vi "SerialNo.vi"() -> (2 "Continue?":bool)   [LabVIEW 2019]
uses:
  globals/QC_RunInformation.vi
panel:
  in  "DB Serial No.:":string
  in  "Device Category:":string(combo)="ATLAS18SS"
  in  "Manufacturer:":string(combo)="Hamamatsu"
  in  "Sensor Serial No.:":string
  in  "Cancel":bool
  in  "OK":bool
  in  "Barcode reader":bool
  # "ATLAS Serial No."
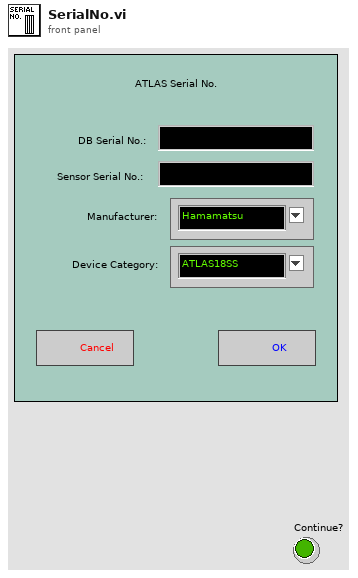
[diagram p1: front panel]
types:
  T1 = cluster{"Institute":string, "Manufacturers":string[], "Devices":string[], "Serialnumbers Lookup DB":string, "Data directory":string, "Backup & screenshot directory":string, "List of known users":string[], "Measurement switch not used":bool, "Measurement Switch":string, "DUT Switch":string}
  T2 = cluster{"Sensor Serial No.:":string, "Wafer Serial No.:":string, "Batch:":string, "Manufacturer:":string, "Device Category:":string, "Database Serial No.:":string, "Date Initiated:":string, "Time Initiated:":string, "Test":string, "Instruments used:":string, "Probeplan used:":string, "End of Run comment:":string, "User:":string}
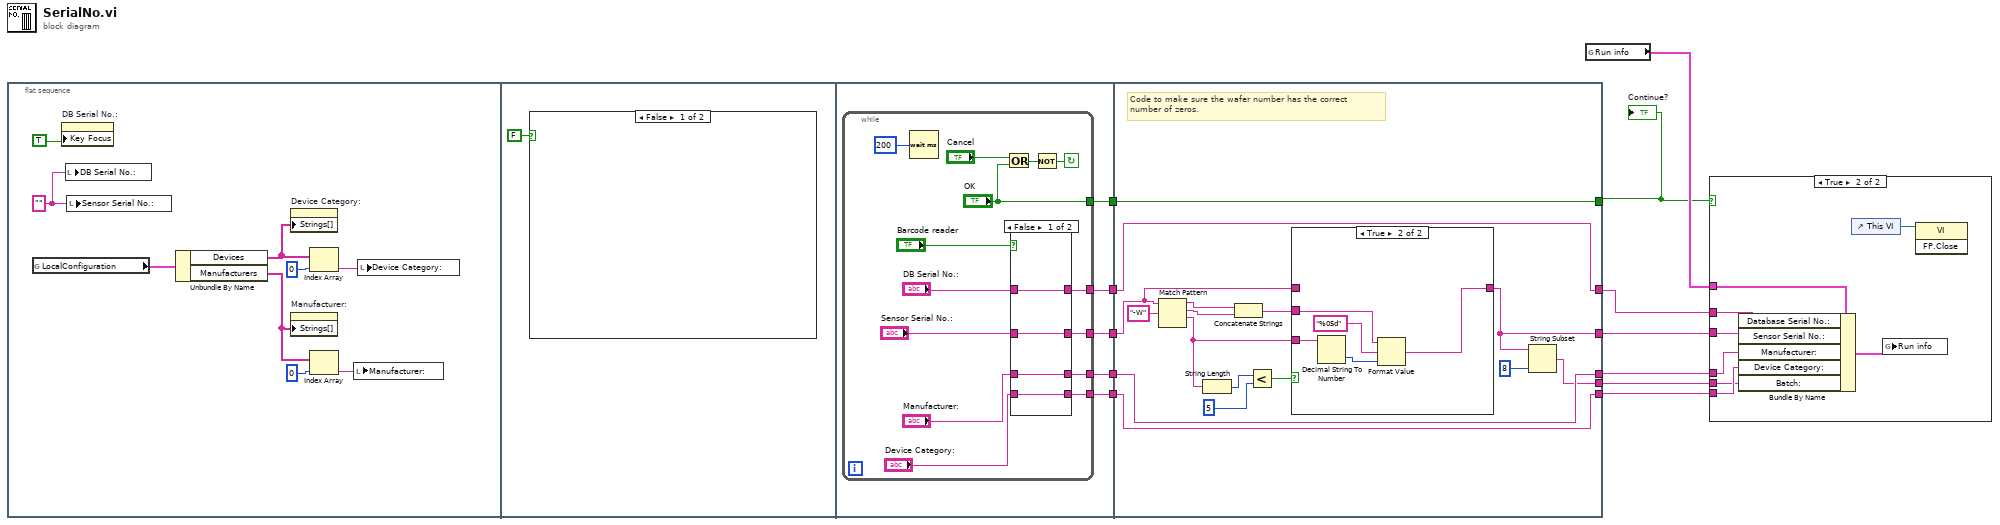
[diagram p0: block diagram]
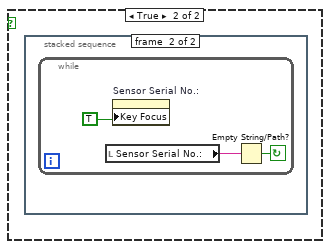
[diagram p3: hidden frame]
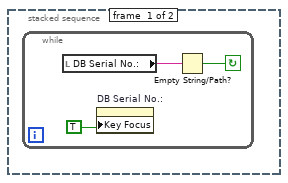
[diagram p4: hidden frame]
diagram:
  n1 = flat-sequence {
    tunnel: [w33] -> w7
    tunnel: [w32] -> w6
    tunnel: [w31] -> w5
    tunnel: [w30] -> w4
    tunnel: [w29] -> w3
    tunnel: [w68] -> w11
    tunnel: [w69] -> w10
    tunnel: [w70] -> w8
    tunnel: [w71] -> w12
    tunnel: w7 -> [w71]
    tunnel: w6 -> [w70]
    tunnel: w5 -> [w69]
    tunnel: w4 -> [w68]
    tunnel: w3 -> [w62]
    tunnel: [w58] -> w2
    tunnel: [w56] -> w1
    frame #0 {
      w21 = ""
      n2 = global read "QC_RunInformation.vi" "LocalConfiguration"() -> (w19:T1)
      n3 = property on="DB Serial No.:" class="Str"("Key Focus"=TRUE) -> ()  [unwired: 2 in, 2 out]
      n4 = local write "DB Serial No.:"(w21) -> ()
      n5 = local write "Sensor Serial No.:"(w21) -> ()
      n6 = Unbundle By Name(w19) -> ("Devices"=w14:string[], "Manufacturers"=w13:string[])
      n7 = property on="Device Category:" class="CmbBox"("Strings[]"=w14) -> ()  [unwired: 2 in, 2 out]
      n8 = property on="Manufacturer:" class="CmbBox"("Strings[]"=w13) -> ()  [unwired: 2 in, 2 out]
      n9 = Index Array(array=w14, index=0) -> (element=w15:string)
      n10 = Index Array(array=w13, index=0) -> (element=w16:string)
      n11 = local write "Manufacturer:"(w16) -> ()
      n12 = local write "Device Category:"(w15) -> ()
    }
    frame #1 {
      n13 = case shown="False" FALSE {
        frame False {
        }
        frame True {
          n14 = stacked-sequence {
            frame #0 {
              n15 = while {
                stop <- w23 continue-if-true
                n16 = local read "DB Serial No.:"() -> (w24:string)
                n17 = property on="DB Serial No.:" class="Str"("Key Focus"=TRUE) -> ()  [unwired: 2 in, 2 out]
                n18 = Empty String/Path?(string/path=w24) -> (empty?=w23:bool)
              }
            }
            frame #1 {
              n19 = while {
                stop <- w27 continue-if-true
                n20 = local read "Sensor Serial No.:"() -> (w26:string)
                n21 = property on="Sensor Serial No.:" class="Str"("Key Focus"=TRUE) -> ()  [unwired: 2 in, 2 out]
                n22 = Empty String/Path?(string/path=w26) -> (empty?=w27:bool)
              }
            }
          }
        }
      }
    }
    frame #2 {
      n23 = while {
        tunnel: ["OK"] -> w32
        tunnel: [w40] -> w29
        tunnel: [w41] -> w33
        tunnel: [w39] -> w31
        tunnel: [w38] -> w30
        stop <- w45 continue-if-true
        n24 = Wait (ms)(milliseconds to wait=200) -> ()  [unwired: 1 out]
        n25 = Or(x="Cancel", y="OK") -> (x .or. y?=w46:bool)
        n26 = case shown="False" "Barcode reader" {
          tunnel: "DB Serial No.:" -> [w51 w55]
          tunnel: "Sensor Serial No.:" -> [w50 w54]
          tunnel: [w51 w55] -> w41
          tunnel: [w50 w54] -> w40
          tunnel: "Manufacturer:" -> [w49 w53]
          tunnel: [w49 w53] -> w39
          tunnel: "Device Category:" -> [w48 w52]
          tunnel: [w48 w52] -> w38
          frame False {
          }
          frame True {
          }
        }
        n27 = Not(x=w46) -> (.not. x?=w45:bool)
      }
    }
    frame #3 {
      # "Code to make sure the wafer number has the correct\nnumber of zeros."
      n28 = Match Pattern(string=w62, regular expression="-W") -> (before substring=w61:string, match substring=w60:string, after substring=w63:string)  [unwired: 1 in, 1 out]
      n29 = String Length(string=w63) -> (length=w66:i32)
      n30 = Concatenate Strings(w61, w60) -> (w59:string)
      n31 = Less?(x=w66, y=5) -> (x < y?=w65:bool)
      n32 = case shown="True" w65 {
        tunnel: w63 -> [_ w77]
        tunnel: w62 -> [w72 _]
        tunnel: [w72 w74] -> w58
        tunnel: w59 -> [_ w76]
        frame False {
        }
        frame True {
          n33 = Decimal String To Number(string=w77) -> (number=w73:i32)  [unwired: 2 in, 1 out]
          n34 = Format Value(string ("")=w76, format string="%05d", value (0)=w73) -> (output string=w74:string)
        }
      }
      n35 = String Subset(string=w58, length (rest)=8 ("length (rest)")) -> (substring=w56:string)  [unwired: 1 in]
    }
  }
  n36 = global read "QC_RunInformation.vi" "Run info"() -> (w9:T2)
  n37 = case shown="True" w8 {
    tunnel: w12 -> [_ w85]
    tunnel: w11 -> [_ w79]
    tunnel: w10 -> [_ w80]
    tunnel: w9 -> [_ w84]
    tunnel: w2 -> [_ w82]
    tunnel: w1 -> [_ w78]
    frame False {
    }
    frame True {
      n38 = Bundle By Name(cluster=w84, "Database Serial No.:"=w85, "Sensor Serial No.:"=w82, "Manufacturer:"=w80, "Device Category:"=w79, "Batch:"=w78) -> (w83:T2)
      n39 = control-ref of="This VI"() -> (w81:refnum<vi>)
      n40 = global write "QC_RunInformation.vi" "Run info"(w83) -> ()
      n41 = invoke class="VI" method="FP.Close"(reference=w81) -> ()  [unwired: 2 in, 3 out]
    }
  }
  "Continue?" <- w8
